vi "Ping.vi"(8 "error in (no error)":errorcluster, 10 "Ping Time":timestamp, 11 "Monitored Actor in":refnum<class "Monitored Actor.lvclass">) -> (0 "error out":errorcluster, 3 "Monitored Actor out":refnum<class "Monitored Actor.lvclass">)   [LabVIEW 2023, in "Monitored Actor.lvlib" / "Monitored Actor.lvclass"]
uses:
  Monitored Actor.lvclass
  C:/Users/Public/Documents/Development/builds/Engine/Actor Framework.lvlibp/1abvi3w/vi.lib/ActorFramework/Actor/Actor.lvclass
  Monitored Actor.lvclass/Monitored Actor.ctl
  Actor Monitor/Actor Monitor Messages/Report Ping Msg/Report Ping Msg.lvclass
  builds/Engine/Actor Framework.lvlibp/1abvi3w/vi.lib/ActorFramework/Actor/Actor.lvclass
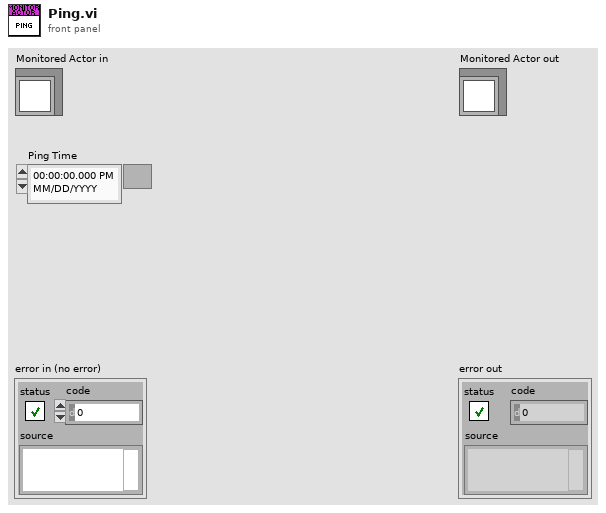
[diagram p1: front panel]
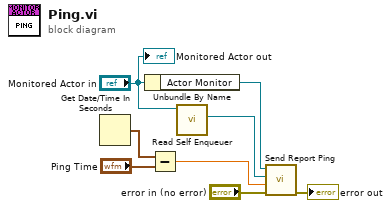
[diagram p0: block diagram]
diagram:
  n1 = Get Date/Time In Seconds() -> (seconds since 1Jan1904=w4:timestamp)
  n2 = Unbundle By Name("Monitored Actor in") -> ("Actor Monitor"=w6:refnum<class "Message Enqueuer.lvclass">)
  n3 = Subtract(x=w4, y="Ping Time") -> (x-y=w3:dbl)
  n4 = call "Read Self Enqueuer.vi"("Actor"="Monitored Actor in") -> ("Self Enqueuer"=w5:refnum<class "Message Enqueuer.lvclass">)  [unwired: 10 in]
  n5 = call "Send Report Ping.vi"("error in (no error)"="error in (no error)", "Ping Duration"=w3, "Actor's Self Q"=w5, "Message Enqueuer in"=w6) -> ("error out"=→"error out":errorcluster)  [unwired: 6 in, 1 out]
  "Monitored Actor out" <- "Monitored Actor in"
